vi "Ilmainfo.vi"() -> (0 "Array":T1)   [LabVIEW 2020]
doc: "Tagastab ilmajaamade järjendi indikaatorina hetkeseisu ilmateenistus.ee andmete järgi erinevates ilmajaamades üle Eesti. Iga ilmajaam omab: nime, temperatuuri, niiskus ja õhurõhku.s"
uses:
  Downloads/visuaalprogrammeerimine/visuaalprogrammeerimine/Ilmajaamad.ctl
  Downloads/visuaalprogrammeerimine/visuaalprogrammeerimine/Ilmajaam.ctl
  <vilib>/xml/Load XML String.vi
  <vilib>/httpClient/LabVIEWHTTPClient.lvlib
  <vilib>/xml/NI_XML.lvlib
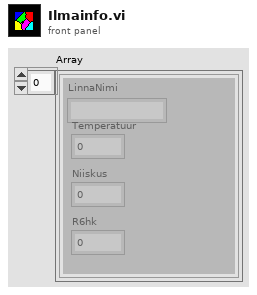
[diagram p1: front panel]
types:
  T1 = typedef "Ilmajaamad.ctl" = T2[]
  T2 = typedef "Ilmajaam.ctl" = cluster{"LinnaNimi":string, "Temperatuur":dbl, "Niiskus":dbl, "R6hk":dbl}
  T3 = typedef "LabVIEWHTTPClient.lvlib/ClientHandle.ctl" = refnum<k1>
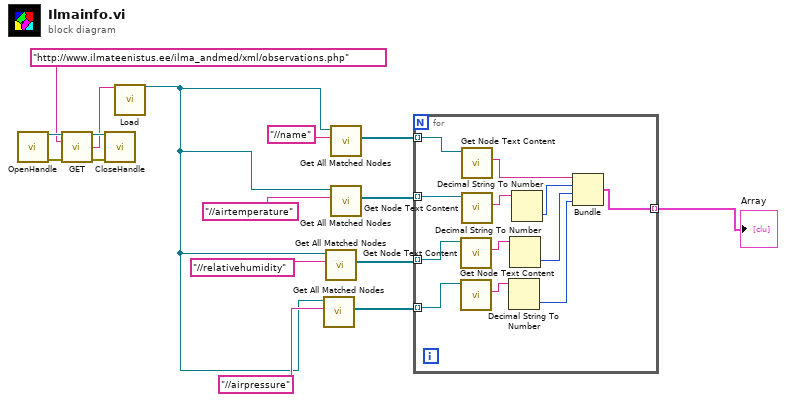
[diagram p0: block diagram]
diagram:
  n1 = call <vilib>:"OpenHandle.vi"() -> ("client handle out"=w16:T3, "error out"=w14:errorcluster)  [unwired: 14 in]
  n2 = call <vilib>:"GET.vi"("client handle"=w16, "url"="http://www.ilmateenistus.ee/ilma_andmed/xml/observations.php", "error in (no error)"=w14) -> ("client handle out"=w15:T3, "body"=w11:string, "error out"=w13:errorcluster)  [unwired: 9 in, 1 out]
  n3 = call <vilib>:"CloseHandle.vi"("client handle"=w15, "error in (no error)"=w13) -> ()  [unwired: 13 in, 1 out]
  n4 = call-poly <vilib>:"Load.vi"("XML string"=w11) -> ("DOM document out"=w2:refnum<k20>)  [unwired: 12 in, 2 out]
  n5 = call <vilib>:"Get All Matched Nodes.vi"("XPath expression"="//airpressure", "node in"=w2) -> ("node result array"=w3:refnum<k20>[])  [unwired: 7 in, 2 out]
  n6 = call <vilib>:"Get All Matched Nodes.vi"("XPath expression"="//relativehumidity", "node in"=w2) -> ("node result array"=w5:refnum<k20>[])  [unwired: 7 in, 2 out]
  n7 = call <vilib>:"Get All Matched Nodes.vi"("XPath expression"="//name", "node in"=w2) -> ("node result array"=w6:refnum<k20>[])  [unwired: 7 in, 2 out]
  n8 = call <vilib>:"Get All Matched Nodes.vi"("XPath expression"="//airtemperature", "node in"=w2) -> ("node result array"=w4:refnum<k20>[])  [unwired: 7 in, 2 out]
  n9 = for {
    tunnel: w6 -> [w28] mode=indexing
    tunnel: w5 -> [w27] mode=indexing
    tunnel: w4 -> [w26] mode=indexing
    tunnel: w3 -> [w25] mode=indexing
    tunnel: [w17] -> w1 mode=indexing
    n10 = call <vilib>:"Get Node Text Content.vi"("node in"=w27) -> ("node text"=w21:string)  [unwired: 8 in, 2 out]
    n11 = call <vilib>:"Get Node Text Content.vi"("node in"=w25) -> ("node text"=w19:string)  [unwired: 8 in, 2 out]
    n12 = call <vilib>:"Get Node Text Content.vi"("node in"=w28) -> ("node text"=w23:string)  [unwired: 8 in, 2 out]
    n13 = call <vilib>:"Get Node Text Content.vi"("node in"=w26) -> ("node text"=w24:string)  [unwired: 8 in, 2 out]
    n14 = Decimal String To Number(string=w19) -> (number=w18:i32)  [unwired: 2 in, 1 out]
    n15 = Decimal String To Number(string=w21) -> (number=w20:i32)  [unwired: 2 in, 1 out]
    n16 = Decimal String To Number(string=w24) -> (number=w22:i32)  [unwired: 2 in, 1 out]
    n17 = Bundle("node text"=w23, w22, w20, w18) -> (w17:cluster{"node text":string, i32, i32, i32})  [unwired: 1 in]
  }
  "Array" <- w1
